vi "Load INI and INIT.vi"(8 "error in (no error)":errorcluster, 11 "configuration file path":path) -> (0 "error out":errorcluster, 3 "Status Connection Out":T1={"Description"="", "Address"="", "Port"=0, "timeout (ms)"=5000, "Termination Character"="\n", "TCP Connection Reference"=refnum, "Open Connection"=FALSE})   [LabVIEW 2017, in "Status Monitor Library.lvlib"]
doc: "Initialising the ini file and opening connection to the tcp port"
uses:
  Status Monitor Library.lvlib
  Communications/Typedefs/DTACQ Connection Data--Cluster.ctl
  Communications/Communications Library.lvlib
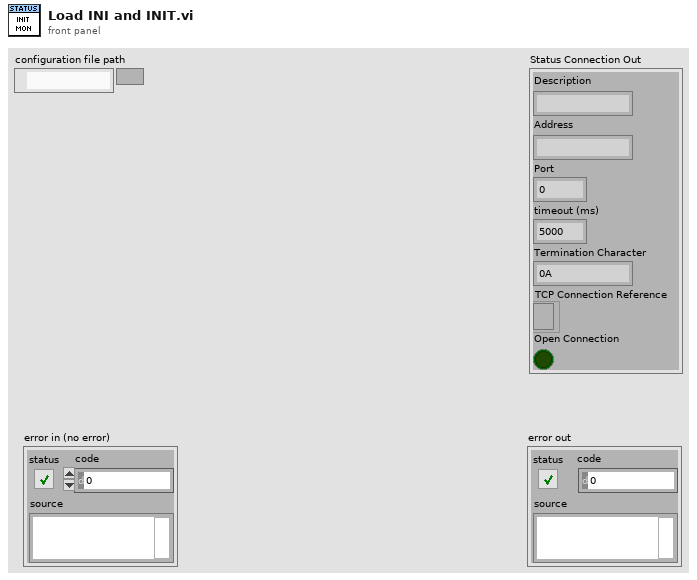
[diagram p1: front panel]
types:
  T1 = typedef "Communications Library.lvlib/DTACQ Connection Data--Cluster.ctl" = cluster{"Description":string, "Address":string, "Port":u16, "timeout (ms)":i32, "Termination Character":string, "TCP Connection Reference":refnum<k5>, "Open Connection":bool}
  T2 = typedef "Communications Library.lvlib/DTACQ Module Carrier Configuration--Cluster.ctl" = cluster{"Name":string, "IP":string, "Control Port":i32, "Timeout (ms)":i32, "Continuous Capture Port (Multiplexed)":i32, "Start HIL Shot Port":i32, "AWG Upload Port (Multiplexed)":i32, "Download Captured Data Port (Multiplexed)":i32, "Module Slots":i32, "Module Configurations":T3[]}
  T3 = typedef "Communications Library.lvlib/DTACQ Module Configuration--Cluster.ctl" = cluster{"Name":string, "Position":string, "Module Type":T4, "Control Port":i32, "Timeout (ms)":i32, "Channels":i32}
  T4 = typedef "Communications Library.lvlib/DTACQ Device Type--Enum.ctl" = enum16{"Carrier", "Analog In Module", "Analog Out Module", "Generic Module"}
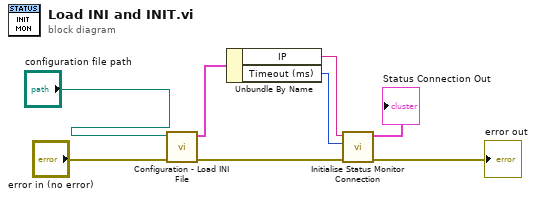
[diagram p0: block diagram]
diagram:
  n1 = call "Configuration - Load INI File.vi"("error in"="error in (no error)", "configuration file path"="configuration file path") -> ("error out"=w4:errorcluster, "Carrier Configuration Out"=w2:T2)  [unwired: 8 in]
  n2 = Unbundle By Name(w2) -> ("IP"=w3:string, "Timeout (ms)"=w5:i32)
  n3 = call "Initialise Status Monitor Connection.vi"("error in"=w4, "timeout (ms)"=w5, "Address"=w3) -> ("error out"=→"error out":errorcluster, "Status Connection Out"=→"Status Connection Out":T1)  [unwired: 7 in]
